vi "CTV.vi"(0 "System no.":i32=1 min=1 max=4 step=1, 2 "Axes to move":string[](array[string]), 3 "Target values":dbl[](array[numeric]) format="%.6f", 4 "No.of digits":i16=4, 5 "error in":errorcluster) -> (19 "error out":errorcluster)   [LabVIEW 2020]
doc: "Set target value for currently selected control mode. A motion induced by CTV can be interrupted by #24, STP or HLT. Servo must be enabled when commanding CTV. No. of digits is the number of digits after the decimal point in the position value(s) that will be sent.\n\nC-413: Motion commands are not allowed when a wave generator is active or the analog input is used for target generation."
panel:
  # "Set target value for currently selected control mode."
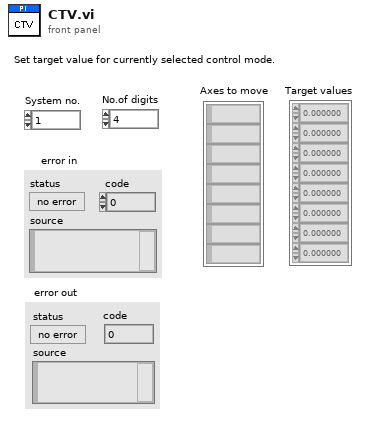
[diagram p1: front panel]
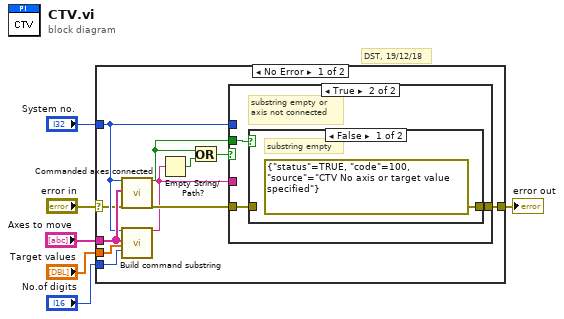
[diagram p0: block diagram]
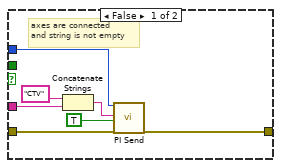
[diagram p2: hidden frame]
diagram:
  # "DST, 19/12/18"
  n1 = case shown="No Error" "error in" {
    selector: "error in" -> [w9 w30]
    tunnel: [w17 w30] -> w6
    tunnel: "Target values" -> [w16 _]
    tunnel: "No.of digits" -> [w15 _]
    tunnel: "System no." -> [w10 _]
    tunnel: "Axes to move" -> [w13 _]
    frame No Error {
      n2 = call "Commanded axes connected.vi"("System no."=w10, "Commanded axes"=w13, "error in"=w9) -> ("Controller error"=w8:bool, "error out"=w14:errorcluster)  [unwired: 1 in, 14 out]
      n3 = call "Build command substring.vi"("System no."=w10, "Affected axes"=w13, "Parameters"=w16, "No. of digits"=w15) -> ("Command substring"=w7:string)  [unwired: 3 in, 12 out]
      n4 = Empty String/Path?(string/path=w7) -> (empty?=w12:bool)
      n5 = Or(x=w8, y=w12) -> (x .or. y?=w11:bool)
      n6 = case shown="True" w11 {
        tunnel: w7 -> [w23 _]
        tunnel: [w19 w27] -> w17
        tunnel: w14 -> [w20 w25]
        tunnel: w8 -> [_ w26]
        tunnel: w10 -> [w18 _]
        frame False {
          # "axes are connected \nand string is not empty"
          n7 = Concatenate Strings("CTV", w23) -> (w21:string)
          n8 = call "PI Send.vi"("System no."=w18, "String to send"=w21, "Attach termination char.?"=TRUE ("Attach Linefeed?"), "error in"=w20) -> ("error out"=w19:errorcluster)  [unwired: 2 in, 13 out]
        }
        frame True {
          # "substring empty or \naxis not connected"
          n9 = case shown="False" w26 {
            tunnel: [errorcluster {"status"=TRUE, "code"=100, "source"="CTV No axis or target value specified"} ("error out") w29] -> w27
            tunnel: w25 -> [_ w29]
            frame False {
              # "substring empty"
            }
            frame True {
              # "commanded axis\nnot connected"
            }
          }
        }
      }
    }
    frame Error {
    }
  }
  "error out" <- w6
